vi "Port Open.vi"(8 "error in (no error)":errorcluster, 11 "AD4212C in":refnum<class "AD4212C.lvclass">) -> (0 "error out":errorcluster, 3 "AD4212C out":refnum<class "AD4212C.lvclass">)   [LabVIEW 2014, in "AD4212C.lvlib" / "AD4212C.lvclass"]
doc: "Abre el puerto COM de la pc colocando el seteado por el usuario y la configuración por defecto que necesita el dispositivo para iniciarse."
uses:
  AD4212C.lvclass
  AD4212C.lvclass/AD4212C.ctl
  API/AD4212C Lib.lvlib
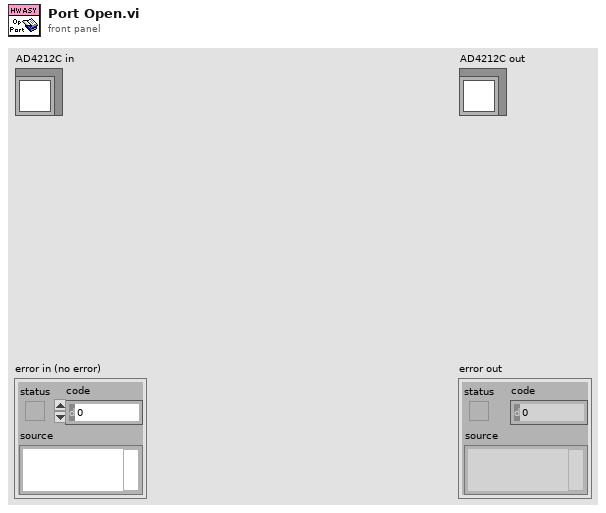
[diagram p1: front panel]
types:
  T1 = typedef "AD4212C Lib.lvlib/Connection Data.ctl" = cluster{"Conection Data":refnum<visa-resource-name>}
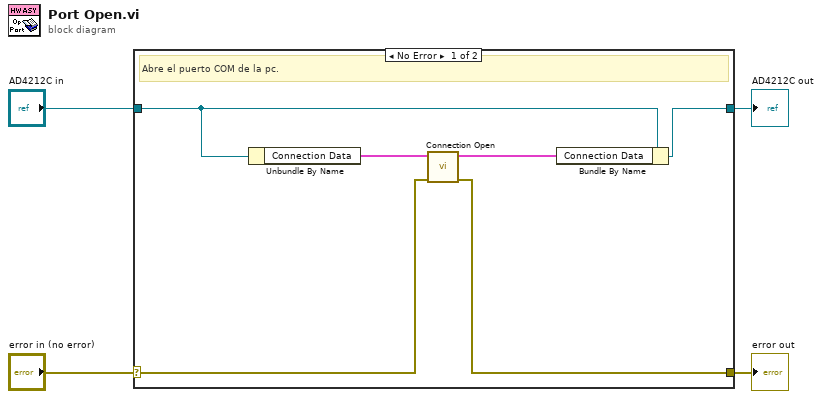
[diagram p0: block diagram]
diagram:
  n1 = case shown="No Error" "error in (no error)" {
    selector: "error in (no error)" -> [w6 w12]
    tunnel: [w5 w12] -> w3
    tunnel: [w7 w11] -> w1
    tunnel: "AD4212C in" -> [w8 w11]
    frame No Error {
      # "Abre el puerto COM de la pc."
      n2 = Unbundle By Name(w8) -> ("Connection Data"=w10:T1)
      n3 = call "Connection Open.vi"("VISA resource name Out 3"=w10, "error in (no error)"=w6) -> ("VISA resource name Out 2"=w9:T1, "error out"=w5:errorcluster)  [unwired: 7 in]
      n4 = Bundle By Name(cluster=w8, "Connection Data"=w9) -> (w7:refnum<class "AD4212C.lvclass">)
    }
    frame Error {
    }
  }
  "error out" <- w3
  "AD4212C out" <- w1
